vi "Patch data preview initialise.vi"(7 "Number of rows to generate":i32, 10 "Dataset path":path, 11 "Scrollbar ref":refnum<vi>) -> (3 "Next state":T3)   [LabVIEW 2020]
uses:
  Typedefs/Patch viewer states.ctl
  Typedefs/Patch viewer internal cluster.ctl
  <vilib>/vision/Image Controls.llb/IMAQ Image.ctl
  Typedefs/Read Write Enum.ctl
  User Interface/Visualisation/Functional Imaging Viewer/SubVIs/Experiment header interface/Typedefs/Header file sections.ctl
  User Interface/Visualisation/Functional Imaging Viewer/SubVIs/Experiment header interface/Typedefs/Header file actions.ctl
panel:
  in  "Start Coordinates":T1(array[cluster])
  in  "Stop Coordinates":T2(array[cluster])
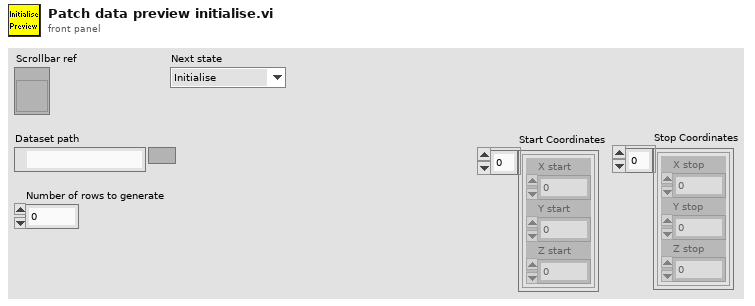
[diagram p1: front panel]
types:
  T1 = cluster{"X start":i32, "Y start":i32, "Z start":i32}[]
  T2 = cluster{"X stop":i32, "Y stop":i32, "Z stop":i32}[]
  T3 = typedef "Patch viewer states.ctl" = enum16{"Initialise", "Refresh", "Idle", "Error"}
  T4 = typedef "Header file actions.ctl" = enum16{"Create", "Open", "Read All", "Read Section", "Write All", "Write Section", "Close"}
  T5 = typedef "Header file sections.ctl" = enum16{"ALL SECTIONS", "LOGIN", "GLOBAL PARAMETERS", "CALIBRATION DATA", "IMAGING MODES", "TIME SERIES", "MOTOR Z-STACK", "AOL Z-STACK", "FUNCTIONAL IMAGING", "VOLUME IMAGING", "MOVEMENT CORRECTION", "CALIBRATION", "STATISTICS", "BIOLOGY INFORMATION"}
  T6 = typedef "Read Write Enum.ctl" = enum16{"Read", "Write"}
  T7 = typedef "Patch viewer internal cluster.ctl" = cluster{"Image ref":T8, "Variable Length ?":bool, "Coordinates of montage positions":cluster{"X\n\nY":i32[]}[], "TDMS refs":refnum<k34>[], "Frames info":cluster{"Frame numbers used":i32[], "Frame position index":i32[]}, "Number of trials":i32, "Cycles in single trial":i32, "Total number of cycles":i32, "Number of patches":i32, "Pixels in a cycle":i32, "Patches info array":cluster{"Pixels in a patch":i32, "X size of patch":i32, "Y size of patch":i32}[], "Start Coordinates":cluster{"X start":i32, "Y start":i32, "Z start":i32}[], "Stop Coordinates":cluster{"X stop":i32, "Y stop":i32, "Z stop":i32}[], "VL Image Refs":T8[], "error":errorcluster}
  T8 = typedef "IMAQ Image.ctl" = refnum<image>
  T9 = cluster{"Pixels in a patch":i32, "X size of patch":i32, "Y size of patch":i32}
  T10 = cluster{"X stop":i32, "Y stop":i32, "Z stop":i32}
  T11 = cluster{"X start":i32, "Y start":i32, "Z start":i32}
  T12 = typedef "Header parameters cluster-ALL.ctl" = cluster{"LOGIN":T13, "GLOBAL PARAMETERS":T14, "IMAGING MODES":T16, "TIME SERIES":T17, "MOTOR Z-STACK ":T20, "AOL Z-STACK":T21, "FUNCTIONAL IMAGING":T22, "VOLUME IMAGING":T22, "MOVEMENT CORRECTION":T26, "CALIBRATION":T28, "STATISTICS":T29, "BIOLOGY INFORMATION":T30, "Calibration Data":T31}
  T13 = typedef "Header params -Login.ctl" = cluster{"User":string, "Profile":string, "Software Version":string, "Experiment Date Time":timestamp}
  T14 = typedef "Header params-Global Parameters.ctl" = cluster{"MicroscopeID":string, "Microscope Type":string, "Objective":string, "Field of View (um)":dbl, "Fill time (us)":dbl, "Experiment Type":T15, "Stimuli Trigger":bool, "Speed Logging":bool}
  T15 = typedef "Experiment Type.ctl" = enum16{"In vivo", "In vitro", "Testing", "Calibration", "Other"}
  T16 = typedef "Header params-Imaging Modes.ctl" = cluster{"Time Series":bool, "Motor Zstack":bool, "AOL Zstack":bool, "Functional Imaging":bool, "Volume Imaging":bool}
  T17 = typedef "Header params-Time Series.ctl" = cluster{"Basic Image meta data":T18, "AOL z":dbl}
  T18 = typedef "Header params-Basic image meta data.ctl" = cluster{"Wavelength (nm)":dbl, "# averaged frames":dbl, "laser power (%)":dbl, "Pockels":dbl, "pixel dwell time (us)":dbl, "pmt 1":dbl, "pmt 2":dbl, "back apperture":dbl, "zoom":dbl, "field of view":dbl, "Frame Size":T19, "AOL x centre":dbl, "AOL y centre":dbl, "Stage x position":dbl, "Stage y position":dbl, "Stage z position":dbl}
  T19 = typedef "Frame Size.ctl" = u16
  T20 = typedef "Header params-Motor Z-stack.ctl" = cluster{"Hdr Basic Image meta data":T18, "Z Start":dbl, "Z Stop":dbl, "No of Planes":i32, "Laser Power (%) at Z Start":dbl, "Laser Power (%) at Z Stop":dbl}
  T21 = typedef "Header params-AOL Z-stack.ctl" = cluster{"Hdr Basic Image meta data":T18, "Z Start":dbl, "Z Stop":dbl, "No of Planes":i32, "Laser Power (%) at Z Start":dbl, "Laser Power (%) at Z Stop":dbl}
  T22 = typedef "Header params-Functional Imaging.ctl" = cluster{"Functional Mode":T23, "Variable Length":bool, "Variable Resolution":bool, "Pockels Modulation":bool, "Stimuli Trigger":bool, "Cool down enabled":bool, "AOL Mode":T24, "Plane Mode":T25, "Miniscan Dwell time per pixel (us)":dbl, "poi dwell time":dbl, "Number of trials":dbl, "Number of cycles":dbl, "Number of pois":dbl, "Number of miniscans":dbl, "Number of pixels in miniscan":dbl, "Rectangle ROI length":dbl, "Rectangle ROI height":dbl, "Frame rate (fps)":dbl, "Acquisition Length":dbl, "video length (sec)":dbl, "Stimuli delay (sec)":dbl, "Cool down time (sec)":dbl, "Basic Image meta data":T18, "Z Start (um)":dbl, "Z Stop (um)":dbl}
  T23 = typedef "Functional Mode.ctl" = enum16{"Point", "Line", "Patch", "Plane", "Volume"}
  T24 = typedef "AOL modes.ctl" = enum16{"Raster", "Structural", "Pointing", "Mini Scan", "Alignment"}
  T25 = typedef "Plane Mode.ctl" = u16
  T26 = typedef "Header params-Movement correction.ctl" = cluster{"Movement Correction":bool, "Axial Reference":bool, "Reference Source":T27, "Full Frame Size":dbl, "Reference Field of View":dbl, "Reference Zoom":dbl, "Reference dwell time (us)":dbl, "Reference X Pixels":dbl, "Reference Y Pixels":dbl, "Number of Z lines":dbl, "Size of Z pixels":dbl, "Axial Pixels":dbl, "Ignore Z lines":dbl, "Reference Scan Cycles":dbl, "Reference Threshold XY":dbl, "Reference Threshold Z":dbl, "Reference Average XY":dbl, "Reference Average Z":dbl, "Proportional Scale":dbl, "Integral Scale":dbl, "Proportional Scale Z":dbl, "Integral Scale Z":dbl, "Diff Threshold":dbl, "Diff Threshold Z":dbl, "Sliding Average":bool, "Reference count reset enabled":bool, "Scan Interval (ms)":dbl, "Ref Plot Refresh Rate (ms)":dbl}
  T27 = typedef "Reference source.ctl" = enum16{"Green channel", "Red channel"}
  T28 = typedef "Header params-Calibration Setup.ctl" = cluster{"Pockels Calibration File":path, "Calibration_ini file":path, "Setup_ini file":path}
  T29 = typedef "Header params-statistics.ctl" = cluster{"Z-stack duration (sec)":dbl, "Number of acquired data-points":dbl, "Acquisition time (ms)":dbl, "Number of acquired frames":dbl, "Intertrial times":dbl[]}
  T30 = typedef "Biology Information.ctl" = cluster{"Animal Code or Name":string, "Animal DoB":string, "Animal Age":string, "Animal Sex":string, "Animal Weight":string, "Date of Injection":string, "Date of Implant":string, "Site of Injection":string, "Animal Ear Notch":string, "AAV constructs":string, "Genetic background":string, "Optical reporter":string, "Region of brain imaged":string, "Other \ncomments":string}
  T31 = typedef "Header params-calibration data.ctl" = cluster{"Objective Name":string, "Calibration Wavelength":dbl, "Sum X":dbl, "Sum Y":dbl, "Diff X":dbl, "Diff Y":dbl, "Distortion Correction":dbl, " Z norm to um Scaling":dbl, " X norm to um Scaling":dbl}
  T32 = cluster{"Frame numbers used":i32[], "Frame position index":i32[]}
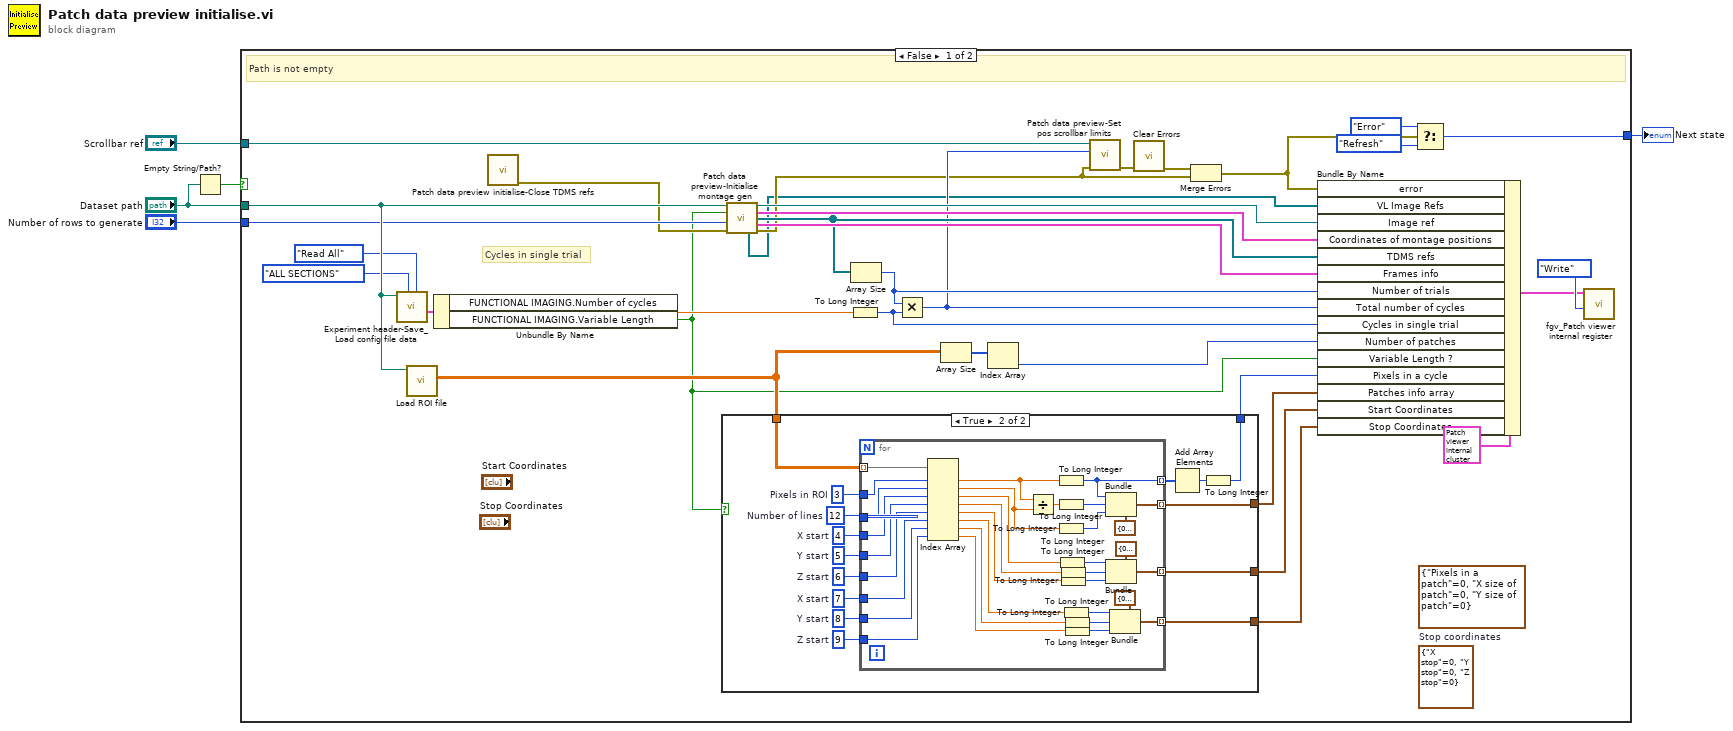
[diagram p0: block diagram]
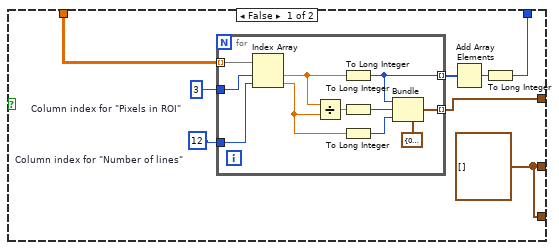
[diagram p2: hidden frame]
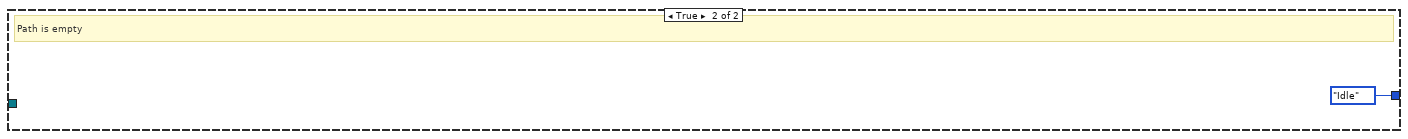
[diagram p3: hidden frame]
diagram:
  n1 = Empty String/Path?(string/path="Dataset path") -> (empty?=w2:bool)
  n2 = case shown="False" w2 {
    tunnel: "Dataset path" -> [w39 _]
    tunnel: "Number of rows to generate" -> [w36 _]
    tunnel: "Scrollbar ref" -> [w29 _]
    tunnel: [w23 Patch_viewer_states."Idle" ("States")] -> w3
    frame False {
      (unwired) T10 {"X stop"=0, "Y stop"=0, "Z stop"=0}  # Stop coordinates
      (unwired) T9 {"Pixels in a patch"=0, "X size of patch"=0, "Y size of patch"=0}
      # "Cycles in single trial"
      # "Path is not empty"
      n3 = call "Experiment header-Save_Load config file data.vi"("Header file actions"=Header_file_actions."Read All", "Header file sections"=Header_file_sections."ALL SECTIONS", "Experiment data folder path"=w39) -> ("All header parameters out"=w35:T12)  [unwired: 7 in, 1 out]
      n4 = call "Load ROI file.vi"("Experiment data folder path"=w39) -> ("ROI Data (header removed)"=w34:dbl[][])  [unwired: 7 in, 3 out]
      n5 = Unbundle By Name(w35) -> ("FUNCTIONAL IMAGING.Number of cycles"=w37:dbl, "FUNCTIONAL IMAGING.Variable Length"=w6:bool)
      n6 = call "Patch data preview initialise-Close TDMS refs.vi"() -> ("error out (no error)"=w22:errorcluster)  [unwired: 11 in]
      n7 = case shown="True" w6 {
        tunnel: w34 -> [w43 w69]
        tunnel: [w42 w68] -> w28
        tunnel: [w41 w67] -> w27
        tunnel: [w40 w60] -> w9
        tunnel: [w40 w59] -> w8
        frame False {
          w40 = T1 []
          w45 = 3  # Column index for "Pixels in ROI"
          w44 = 12  # Column index for "Number of lines"
          n8 = for {
            tunnel: w43 -> [w58] mode=indexing
            tunnel: w45 -> [w57]
            tunnel: w44 -> [w56]
            tunnel: [w53] -> w42 mode=indexing
            tunnel: [w48] -> w47 mode=indexing
            n9 = Index Array(array=w58, index #1=w57, index #2=w56) -> (element #1=w52:dbl, element #2=w54:dbl)
            n10 = Divide(x=w52, y=w54) -> (x/y=w55:dbl)
            n11 = To Long Integer(number=w52) -> (32bit integer=w48:i32)
            n12 = To Long Integer(number=w55) -> (32bit integer=w49:i32)
            n13 = To Long Integer(number=w54) -> (32bit integer=w50:i32)
            n14 = Bundle(cluster=T9 {"Pixels in a patch"=0, "X size of patch"=0, "Y size of patch"=0}, "Pixels in a patch"=w48, "X size of patch"=w49, "Y size of patch"=w50) -> (w53:T9)
          }
          n15 = Add Array Elements(numeric array=w47) -> (sum=w46:i32)
          n16 = To Long Integer(number=w46) -> (32bit integer=w41:i32)
        }
        frame True {
          w61 = 9  # Z start
          w62 = 8  # Y start
          w63 = 7  # X start
          w64 = 6  # Z start
          w65 = 5  # Y start
          w66 = 4  # X start
          w71 = 3  # Pixels in ROI
          w70 = 12  # Number of lines
          n17 = for {
            tunnel: w69 -> [w106] mode=indexing
            tunnel: w71 -> [w105]
            tunnel: w70 -> [w104]
            tunnel: [w101] -> w68 mode=indexing
            tunnel: [w96] -> w73 mode=indexing
            tunnel: w66 -> [w95]
            tunnel: w65 -> [w94]
            tunnel: w64 -> [w93]
            tunnel: w63 -> [w92]
            tunnel: w62 -> [w91]
            tunnel: w61 -> [w90]
            tunnel: [w82] -> w60 mode=indexing
            tunnel: [w74] -> w59 mode=indexing
            n18 = Index Array(array=w106, index #1=w105, index #2=w104, index #3=w95, index #4=w94, index #5=w93, index #6=w92, index #7=w91, index #8=w90) -> (element #1=w100:dbl, element #2=w102:dbl, element #3=w88:dbl, element #4=w86:dbl, element #5=w83:dbl, element #6=w77:dbl, element #7=w76:dbl, element #8=w75:dbl)
            n19 = Divide(x=w100, y=w102) -> (x/y=w103:dbl)
            n20 = To Long Integer(number=w100) -> (32bit integer=w96:i32)
            n21 = To Long Integer(number=w103) -> (32bit integer=w97:i32)
            n22 = To Long Integer(number=w102) -> (32bit integer=w98:i32)
            n23 = To Long Integer(number=w88) -> (32bit integer=w87:i32)
            n24 = To Long Integer(number=w86) -> (32bit integer=w85:i32)
            n25 = To Long Integer(number=w83) -> (32bit integer=w84:i32)
            n26 = To Long Integer(number=w77) -> (32bit integer=w81:i32)
            n27 = To Long Integer(number=w76) -> (32bit integer=w80:i32)
            n28 = To Long Integer(number=w75) -> (32bit integer=w79:i32)
            n29 = Bundle(cluster=T9 {"Pixels in a patch"=0, "X size of patch"=0, "Y size of patch"=0}, "Pixels in a patch"=w96, "X size of patch"=w97, "Y size of patch"=w98) -> (w101:T9)
            n30 = Bundle(cluster=T11 {"X start"=0, "Y start"=0, "Z start"=0}, "X start"=w87, "Y start"=w85, "Z start"=w84) -> (w82:T11)
            n31 = Bundle(cluster=T10 {"X stop"=0, "Y stop"=0, "Z stop"=0} ("Stop coordinates"), "X stop"=w81, "Y stop"=w80, "Z stop"=w79) -> (w74:T10)
          }
          n32 = Add Array Elements(numeric array=w73) -> (sum=w72:i32)
          n33 = To Long Integer(number=w72) -> (32bit integer=w67:i32)
        }
      }
      n34 = call "Patch data preview-Initialise montage gen.vi"("ExperimentPath"=w39, "Variable length"=w6, "error in (no error)"=w22, "Number of rows to generate"=w36) -> ("Image ref (Montage)"=w30:T8, "Coordinates of montage positions"=w31:cluster{"X\n\nY":i32[]}[], "TDMS references(All Trials)"=w21:refnum<k34>[], "Frames info"=w32:T32, "VL Image Refs"=w7:T8[], "error out"=w13:errorcluster)  [unwired: 5 in, 1 out]
      n35 = To Long Integer(number=w37) -> (32bit integer=w20:i32)
      n36 = Array Size(array=w21) -> (size(s)=w19:i32)
      n37 = Multiply(x=w19, y=w20) -> (x*y=w16:i32)
      n38 = Array Size(array=w34) -> (size(s)=w38:i32[])
      n39 = Index Array(array=w38) -> (element=w26:i32)  [unwired: 1 in]
      n40 = call "Patch data preview-Set pos scrollbar limits.vi"("error in (no error)"=w13, "Last cycle's number"=w16, "Scrollbar"=w29) -> ("error out"=w15:errorcluster)  [unwired: 7 in, 1 out]
      n41 = call <vilib>:"Clear Errors.vi"("error in (no error)"=w15) -> ("error out"=w14:errorcluster)  [unwired: 5 in, 1 out]
      n42 = Merge Errors(w14, w13) -> (w12:errorcluster)
      n43 = Bundle By Name(cluster=T7 {"Image ref"=refnum, "Variable Length ?"=FALSE, "Coordinates of montage positions"=[], "TDMS refs"=[], "Frames info"={"Frame numbers used"=[], "Frame position index"=[]}, "Number of trials"=0, "Cycles in single trial"=0, "Total number of cycles"=0, "Number of patches"=0, "Pixels in a cycle"=0, "Patches info array"=[], "Start Coordinates"=[], "Stop Coordinates"=[], "VL Image Refs"=[], "error"={"status"=FALSE, "code"=0, "source"=""}} ("Register cluster"), "error"=w12, "VL Image Refs"=w7, "Image ref"=w30, "Coordinates of montage positions"=w31, "TDMS refs"=w21, "Frames info"=w32, "Number of trials"=w19, "Total number of cycles"=w16, "Cycles in single trial"=w20, "Number of patches"=w26, "Variable Length ?"=w6, "Pixels in a cycle"=w27, "Patches info array"=w28, "Start Coordinates"=w9, "Stop Coordinates"=w8) -> (w17:T7)
      n44 = Select(t=Patch_viewer_states."Error" ("States"), s=w12, f=Patch_viewer_states."Refresh" ("States")) -> (s? t:f=w23:T3)
      n45 = call "fgv_Patch viewer internal register.vi"("Function"=Read_Write_Enum."Write", "Registered setup"=w17) -> ()  [unwired: 9 in, 1 out]
    }
    frame True {
      # "Path is empty"
    }
  }
  "Next state" <- w3
